vi "wait_for_value.vi"(9 "error in":errorcluster, 10 "anything":variant) -> (1 "error out":errorcluster)   [LabVIEW 2015]
doc: "This vi can be used for flow controll by delaying the error line untill this vi recieves an input"
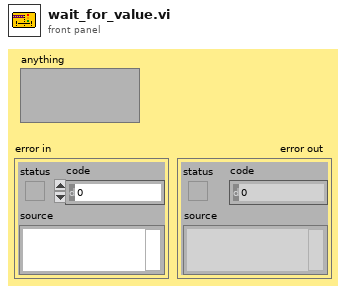
[diagram p1: front panel]
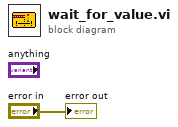
[diagram p0: block diagram]
diagram:
  "error out" <- "error in"
